vi "Demo - Transient Capture (Multiple Shots)_for_sub_panel.vi"(6 "Soft Trigger":bool=TRUE, 9 "Post-Trigger Samples":i32=100000, 10 "Pre-Trigger Samples":i32, 11 "configuration file path":path) -> ()   [LabVIEW 2017]
doc: "Demonstration of transient capture mode, in a continuos loop"
uses:
  Communications/Communications Library.lvlib
panel:
  in  "stop":bool
  in  "ARM":bool
  out "Waveform Graph":i16[][](graph)
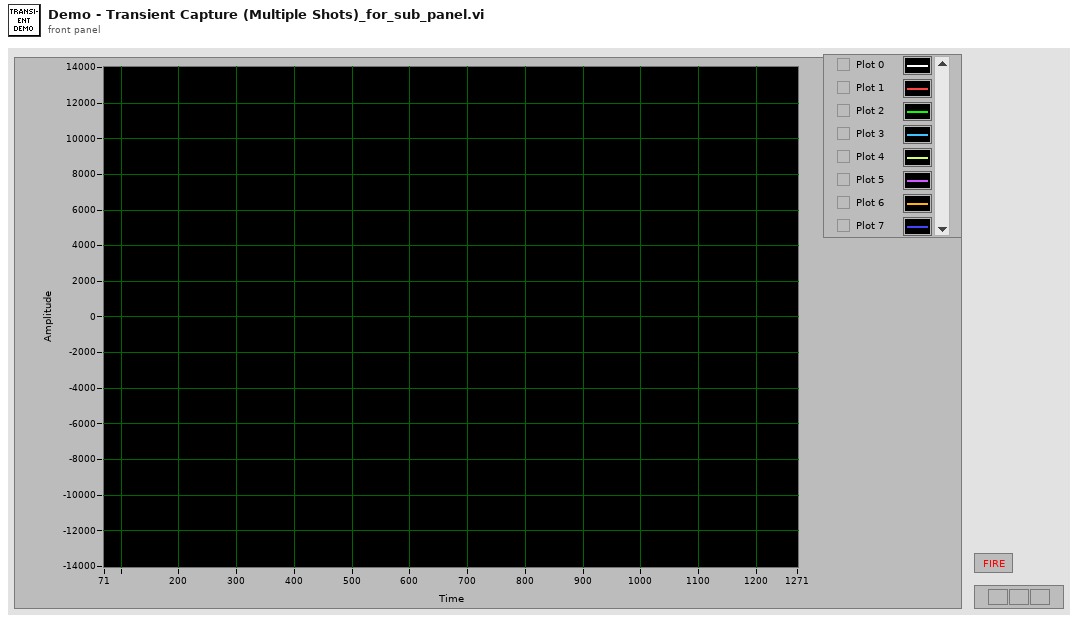
[diagram p1: front panel]
types:
  T1 = typedef "Communications Library.lvlib/DTACQ Module Carrier Configuration--Cluster.ctl" = cluster{"Name":string, "IP":string, "Control Port":i32, "Timeout (ms)":i32, "Continuous Capture Port (Multiplexed)":i32, "Start HIL Shot Port":i32, "AWG Upload Port (Multiplexed)":i32, "Download Captured Data Port (Multiplexed)":i32, "Module Slots":i32, "Module Configurations":T2[]}
  T2 = typedef "Communications Library.lvlib/DTACQ Module Configuration--Cluster.ctl" = cluster{"Name":string, "Position":string, "Module Type":T3, "Control Port":i32, "Timeout (ms)":i32, "Channels":i32}
  T3 = typedef "Communications Library.lvlib/DTACQ Device Type--Enum.ctl" = enum16{"Carrier", "Analog In Module", "Analog Out Module", "Generic Module"}
  T4 = typedef "Communications Library.lvlib/DTACQ Connection Data--Cluster.ctl" = cluster{"Description":string, "Address":string, "Port":u16, "timeout (ms)":i32, "Termination Character":string, "TCP Connection Reference":refnum<k5>, "Open Connection":bool}
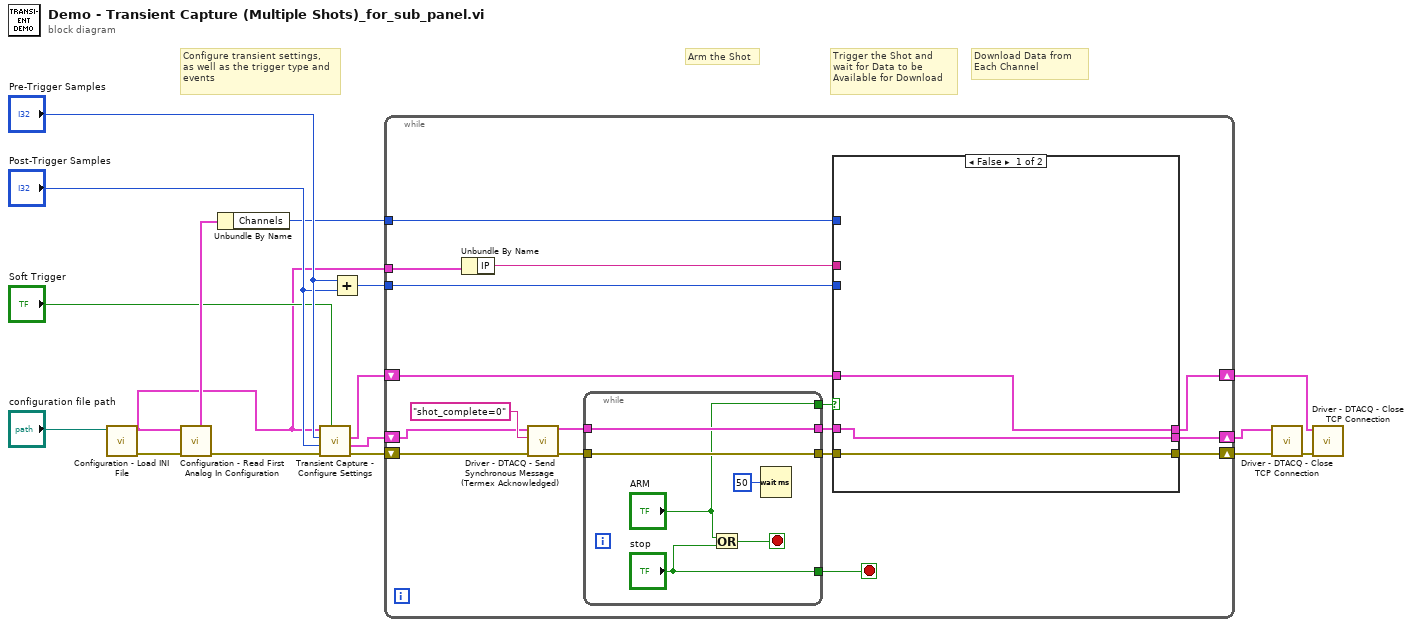
[diagram p0: block diagram]
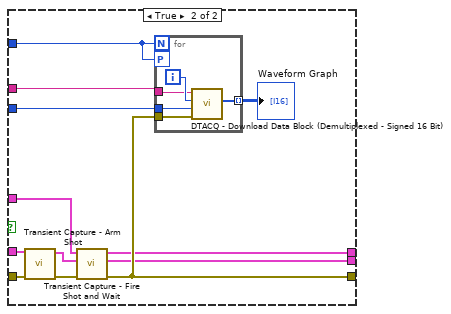
[diagram p2: hidden frame]
diagram:
  # "Configure transient settings,\nas well as the trigger type and\nevents"
  # "Trigger the Shot and\nwait for Data to be\nAvailable for Download"
  # "Download Data from \nEach Channel"
  # "Arm the Shot"
  n1 = call "Configuration - Load INI File.vi"("configuration file path"="configuration file path") -> ("error out"=w13:errorcluster, "Carrier Configuration Out"=w3:T1)  [unwired: 9 in]
  n2 = call "Configuration - Read First Analog In Configuration.vi"("error in"=w13, "Carrier Configuration"=w3) -> ("error out"=w12:errorcluster, "AI - Module Configuration"=w14:T2)  [unwired: 5 in, 3 out]
  n3 = Unbundle By Name(w14) -> ("Channels"=w6:i32)
  n4 = call "Transient Capture - Configure Settings.vi"("Soft Trigger"="Soft Trigger", "error in"=w12, "Samples to Read (Post Trigger)"="Post-Trigger Samples", "Samples to Read (Pre Trigger)"="Pre-Trigger Samples", "Carrier Configuration"=w3) -> ("error out"=w10:errorcluster, "Carrier Connection Out"=w5:T4, "AI Connection Out"=w4:T4)  [unwired: 4 in]
  n5 = Add(x="Pre-Trigger Samples", y="Post-Trigger Samples") -> (x+y=w9:i32)
  n6 = while {
    tunnel: w3 -> [w20]
    tunnel: w9 -> [w33]
    tunnel: w6 -> [w26]
    shift-right: [w32] -> w8
    shift-left: w10 -> [w24]
    shift-right: [w31] -> w1
    shift-left: w4 -> [w28]
    shift-right: [w30] -> w2
    shift-left: w5 -> [w23]
    stop <- w27 stop-if-true
    n7 = Unbundle By Name(w20) -> ("IP"=w19:string)
    n8 = call "Driver - DTACQ - Send Synchronous Message (Termex Acknowledged).vi"("error in"=w24, "Message to Send"="shot_complete=0", "DTACQ Connection Data In"=w23) -> ("error out"=w22:errorcluster, "DTACQ Connection Data Out"=w21:T4)  [unwired: 5 in, 2 out]
    n9 = while {
      tunnel: [w57] -> w34
      tunnel: [w56] -> w29
      tunnel: ["stop"] -> w27
      tunnel: w22 -> [w57]
      tunnel: w21 -> [w56]
      tunnel: ["ARM"] -> w18
      stop <- w59 stop-if-true
      n10 = Or(x="ARM", y="stop") -> (x .or. y?=w59:bool)
      n11 = Wait (ms)(milliseconds to wait=u32 50) -> ()  [unwired: 1 out]
    }
    n12 = case shown="False" w18 {
      tunnel: w34 -> [w36 w48]
      tunnel: w33 -> [_ w46]
      tunnel: [w36 w45] -> w32
      tunnel: [w35 w44] -> w31
      tunnel: [w37 w43] -> w30
      tunnel: w29 -> [w37 w42]
      tunnel: w28 -> [w35 w40]
      tunnel: w26 -> [_ w39]
      tunnel: w19 -> [_ w38]
      frame False {
      }
      frame True {
        n13 = call "Transient Capture - Arm Shot.vi"("error in"=w48, "Carrier Connection In"=w42) -> ("error out"=w47:errorcluster, "DTACQ Connection Out"=w41:T4)  [unwired: 8 in]
        n14 = call "Transient Capture - Fire Shot and Wait.vi"("error in"=w47, "Carrier Connection In"=w41, "AI Connection In"=w40) -> ("error out"=w45:errorcluster, "Carrier Connection Out"=w43:T4, "AI Connection Out"=w44:T4)  [unwired: 6 in]
        n15 = for {
          N: w39 -> [_]
          tunnel: [w53] -> w49 mode=indexing
          tunnel: w46 -> [w52]
          tunnel: w38 -> [w51]
          tunnel: w45 -> [w50]
          workers-P: w39 -> [_]
          i -> [w54]
          n16 = call "DTACQ - Download Data Block (Demultiplexed - Signed 16 Bit).vi"("error in"=w50, "Maximum Number of Samples"=w52, "Channel Number"=w54, "Address"=w51) -> ("(Signed) 16 Bit Array"=w53:i16[])  [unwired: 5 in, 2 out]
        }
        "Waveform Graph" <- w49
      }
    }
  }
  n17 = call "Driver - DTACQ - Close TCP Connection.vi"("error in"=w8, "DTACQ Connection Data In"=w2) -> ("error out"=w7:errorcluster)  [unwired: 8 in, 1 out]
  n18 = call "Driver - DTACQ - Close TCP Connection.vi"("error in"=w7, "DTACQ Connection Data In"=w1) -> ()  [unwired: 8 in, 2 out]
